vi "SQL_Table_Unit_Test_Gear_System_Insert.vi"(10 "时间标识":timestamp, 11 "齿轮子系统数据":T1) -> (3 "error out":errorcluster)   [LabVIEW 2014]
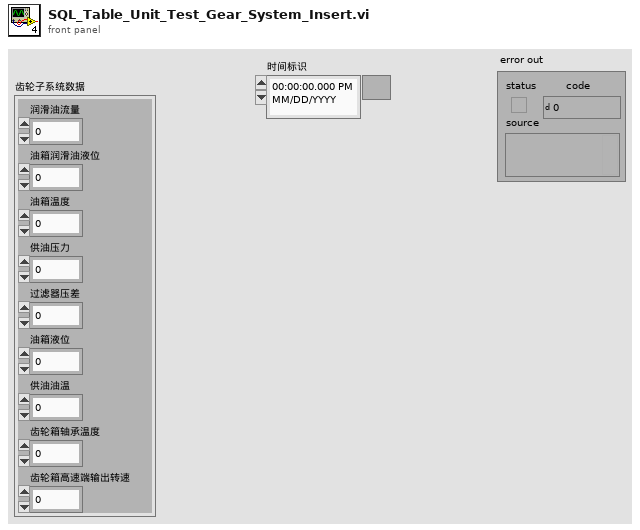
[diagram p1: front panel]
types:
  T1 = cluster{"润滑油流量":u16, "油箱润滑油液位":u16, "油箱温度":u16, "供油压力":u16, "过滤器压差":u16, "油箱液位":u16, "供油油温":u16, "齿轮箱轴承温度":u16, "齿轮箱高速端输出转速":u16}
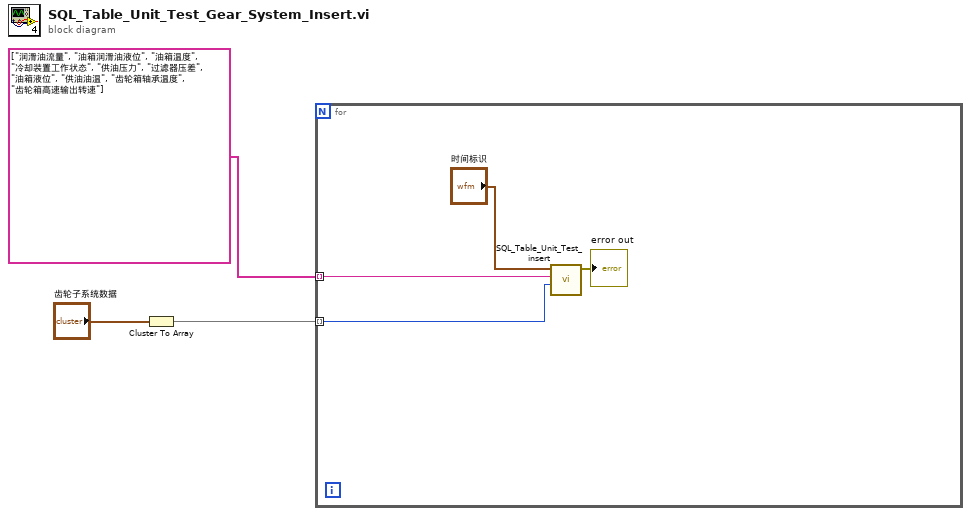
[diagram p0: block diagram]
diagram:
  n1 = Cluster To Array(cluster="齿轮子系统数据") -> (array=w2:u16[])
  n2 = for {
    tunnel: string[] ["润滑油流量", "油箱润滑油液位", "油箱温度", "冷却装置工作状态", "供油压力", "过滤器压差", "油箱液位", "供油油温", "齿轮箱轴承温度", "齿轮箱高速输出转速"] -> [w6] mode=indexing
    tunnel: w2 -> [w5] mode=indexing
    n3 = call "SQL_Table_Unit_Test_insert.vi"("数据数值"=w5, "数据名称"=w6, "时间标识"="时间标识") -> ("error out"=→"error out":errorcluster)  [unwired: 8 in]
  }
